vi "Finish.vi"(8 "Error In":errorcluster, 11 "Parser In":refnum<class "Parser.lvclass">) -> (0 "Error Out":errorcluster, 3 "Parser Out":refnum<class "Parser.lvclass">)   [LabVIEW 2018, in "Toolkit.lvlib" / "Parser.lvclass"]
uses:
  Parser.lvclass
  Parser.lvclass/Parser.ctl
  Tokens/Text/Text.lvclass
  D:/Users/cfield/Code/Field R&D Services/Mustache/trunk/src/Mustache/Public/Tokens/Public/Abstract/Abstract.lvclass
  Tokens/EscapedVariable/EscapedVariable.lvclass
  D:/Users/cfield/Code/Field R&D Services/Mustache/trunk/src/Mustache/Public/Tokens/Public/Keyable/Keyable.lvclass
  Tokens/UnescapedVariable/UnescapedVariable.lvclass
  Tokens/BeginSection/BeginSection.lvclass
  Tokens/InvertedSection/InvertedSection.lvclass
  Tokens/EndSection/EndSection.lvclass
  Tokens/Partial/Partial.lvclass
  Tokens/Keyable/API/Keyable.lvclass
  Tokens/Text/API/New.vi
  <vilib>/Utility/error.llb/Trim Whitespace.vi
  Tokens/EscapedVariable/API/New.vi
  Tokens/UnescapedVariable/API/New.vi
  Tokens/BeginSection/API/New.vi
  Tokens/InvertedSection/API/New.vi
  Tokens/EndSection/API/New.vi
  Tokens/Partial/API/New.vi
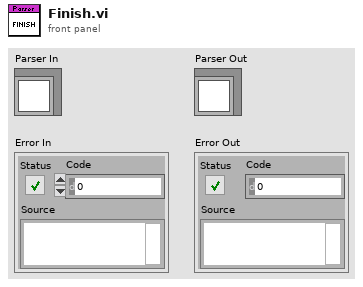
[diagram p1: front panel]
types:
  T1 = typedef "Toolkit.lvlib/Parser.lvclass/States.ctl" = enum16{"Text", "Open Delimiter", "Tag Type", "Tag Key", "Close Delimiter"}
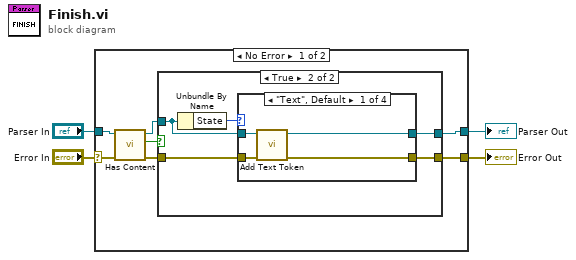
[diagram p0: block diagram]
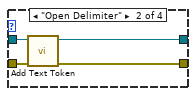
[diagram p3: hidden frame]
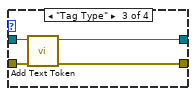
[diagram p4: hidden frame]
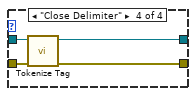
[diagram p5: hidden frame]
diagram:
  n1 = case shown="No Error" "Error In" {
    selector: "Error In" -> [w5 w35]
    tunnel: [w11 w36] -> w4
    tunnel: "Parser In" -> [w7 w36]
    tunnel: [w6 w35] -> w2
    frame No Error {
      n2 = call "Has Content.vi"("Error In"=w5, "Parser In"=w7) -> ("Error Out"=w10:errorcluster, "Content"=w8:bool, "Parser Out"=w9:refnum<class "Parser.lvclass">)  [unwired: 7 in]
      n3 = case shown="True" w8 {
        tunnel: w9 -> [w12 w17]
        tunnel: w10 -> [w13 w16]
        tunnel: [w12 w15] -> w11
        tunnel: [w13 w14] -> w6
        frame False {
        }
        frame True {
          n4 = Unbundle By Name(w17) -> ("State"=w18:T1)
          n5 = case shown="\"Text\", Default" w18 {
            tunnel: w17 -> [w22 w26 w30 w34]
            tunnel: w16 -> [w21 w23 w27 w31]
            tunnel: [w20 w24 w28 w32] -> w14
            tunnel: [w19 w25 w29 w33] -> w15
            frame "Text", Default {
              n6 = call "Add Text Token.vi"("Error In"=w21, "Parser In"=w22) -> ("Error Out"=w20:errorcluster, "Parser Out"=w19:refnum<class "Parser.lvclass">)  [unwired: 8 in]
            }
            frame "Open Delimiter" {
              n7 = call "Add Text Token.vi"("Error In"=w23, "Parser In"=w26) -> ("Error Out"=w24:errorcluster, "Parser Out"=w25:refnum<class "Parser.lvclass">)  [unwired: 8 in]
            }
            frame "Tag Type" {
              n8 = call "Add Text Token.vi"("Error In"=w27, "Parser In"=w30) -> ("Error Out"=w28:errorcluster, "Parser Out"=w29:refnum<class "Parser.lvclass">)  [unwired: 8 in]
            }
            frame "Close Delimiter" {
              n9 = call "Tokenize Tag.vi"("Error In"=w31, "Parser In"=w34) -> ("Error Out"=w32:errorcluster, "Parser Out"=w33:refnum<class "Parser.lvclass">)  [unwired: 8 in]
            }
          }
        }
      }
    }
    frame Error {
    }
  }
  "Parser Out" <- w4
  "Error Out" <- w2
